vi "Servo Motor Emulator.vi"(10 "Servo Motor Emulator Queue in":refnum<queue>, 11 "Device Manager Queue in":refnum<queue>) -> (0 "error out":errorcluster)   [LabVIEW 2026]
uses:
  support/Message Queue/Message Cluster.ctl
  controls/Servo Controller Private Data.ctl
  support/Message Queue/Enqueue Message (Single).vi
  <vilib>/Utility/error.llb/Error Cluster From Error Code.vi
  <vilib>/ErrorRing/Error Ring.xnode
  support/Message Queue/Message Queue.lvlib
  support/User Event - Stop/User Event - Stop.lvlib
panel:
  in  "RH":dbl
  in  "Temperature":dbl
  out "Position":dbl(knob) scale=0.0..180.0
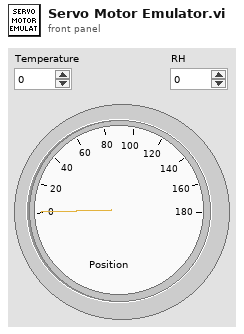
[diagram p1: front panel]
types:
  T1 = typedef "Servo Controller Private Data.ctl" = cluster{"Placeholder":bool}
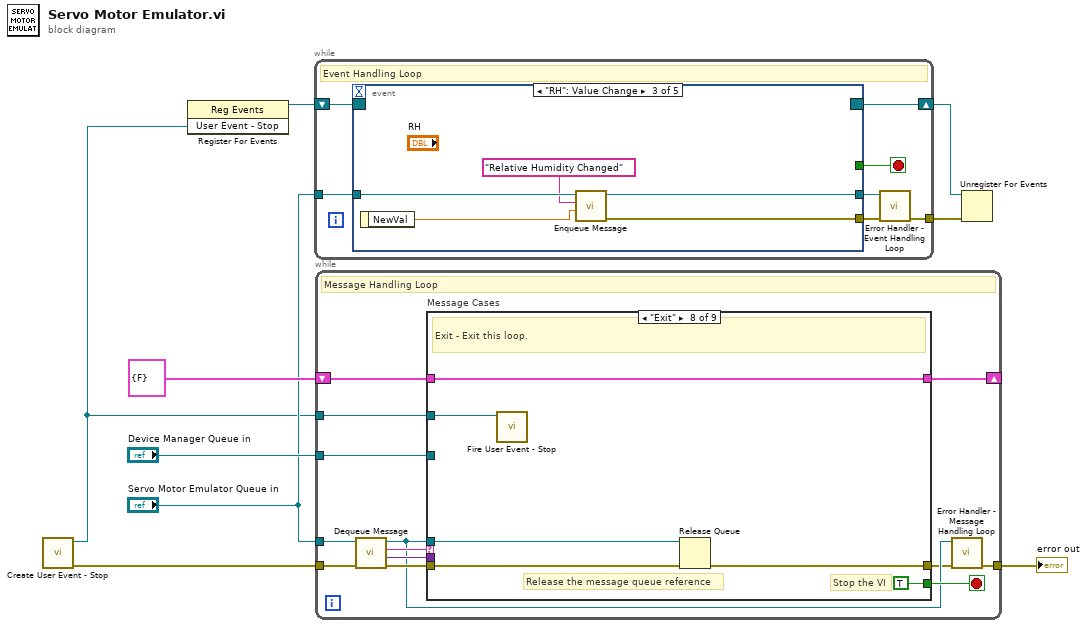
[diagram p0: block diagram]
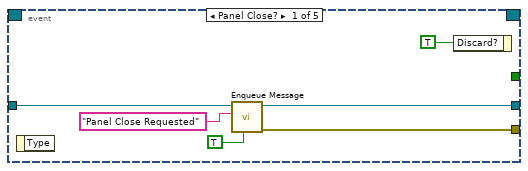
[diagram p2: hidden frame]
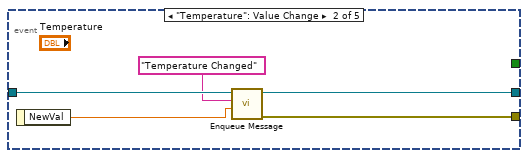
[diagram p3: hidden frame]
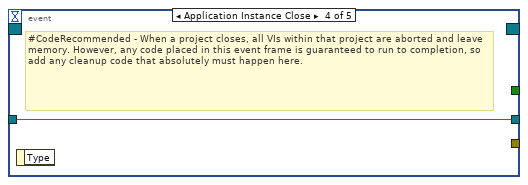
[diagram p4: hidden frame]
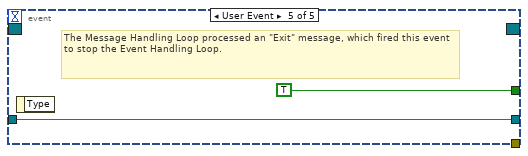
[diagram p5: hidden frame]
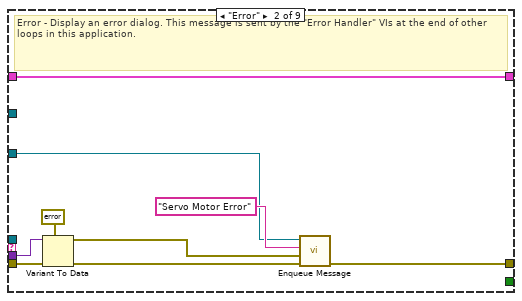
[diagram p7: hidden frame]
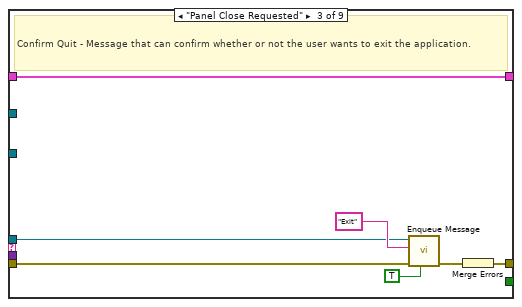
[diagram p8: hidden frame]
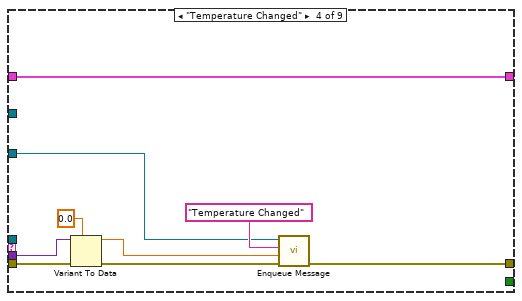
[diagram p9: hidden frame]
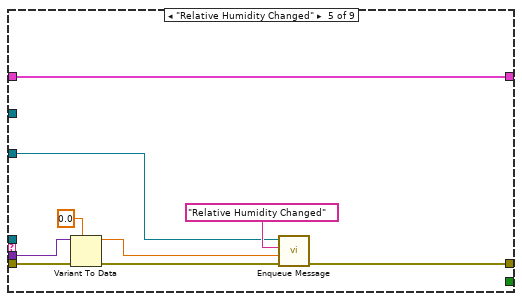
[diagram p10: hidden frame]
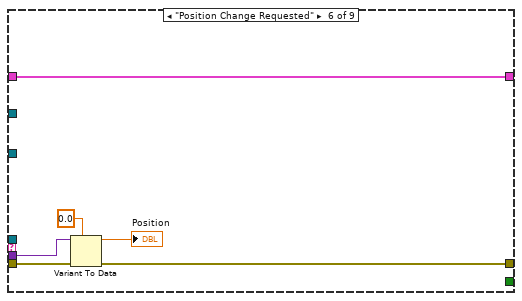
[diagram p11: hidden frame]
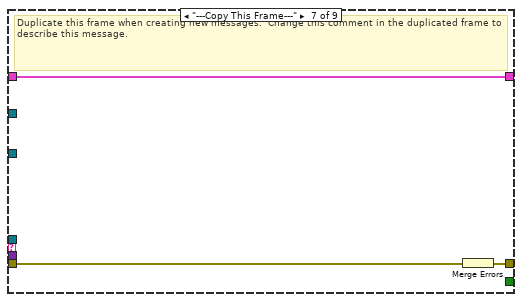
[diagram p12: hidden frame]
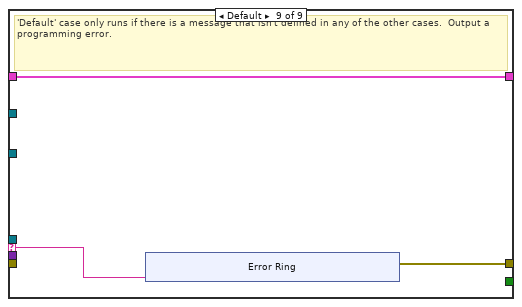
[diagram p13: hidden frame]
diagram:
  n1 = call "Create User Event - Stop.vi"() -> ("error out"=w3:errorcluster, "User Event - Stop"=w1:refnum<user-event>)  [unwired: 10 in]
  n2 = register-events(w1) -> (reference out=w4:refnum<event-registration>)  [unwired: 2 in, 1 out]
  n3 = while {
    tunnel: "Servo Motor Emulator Queue in" -> [w16]
    shift-right: [w14] -> w6
    shift-left: w4 -> [w15]
    tunnel: [w10] -> w5
    stop <- w12 stop-if-true
    # "Event Handling Loop"
    n4 = event shown="[2] \"RH\": Value Change" {
      selector: w15 -> [_ _ _ _ _]
      dyn-events: [_ _ _ _ _] -> w14
      timeout: _ -> [_ _ _ _ _]
      tunnel: [_ _ _ _ TRUE ("Discard?")] -> w12
      tunnel: w16 -> [w21 w27 w32 w33 w35]
      tunnel: [w20 w26 w31 _ _] -> w13
      tunnel: [w19 w25 w30 w33 w35] -> w11
      event Panel Close? {
        n5 = event-data() -> ()  [unwired: 1 in, 1 out]
        n6 = call-poly "Enqueue Message.vi"("Priority Message? (F)"=TRUE, "Message"="Panel Close Requested", "Message Queue"=w21) -> ("error out"=w20:errorcluster, "dup Message Queue"=w19:refnum<queue>)  [unwired: 7 in]
        n7 = event-data("Discard?"=TRUE) -> ()  [unwired: 1 in, 1 out]
      }
      event "Temperature": Value Change {
        n8 = event-data() -> ("NewVal"=w23:dbl)  [unwired: 1 in]
        n9 = call-poly "Enqueue Message.vi"("Message Data"=w23, "Message"="Temperature Changed", "Message Queue"=w27) -> ("error out"=w26:errorcluster, "dup Message Queue"=w25:refnum<queue>)  [unwired: 7 in]
      }
      event "RH": Value Change {
        n10 = event-data() -> ("NewVal"=w28:dbl)  [unwired: 1 in]
        n11 = call-poly "Enqueue Message.vi"("Message Data"=w28, "Message"="Relative Humidity Changed", "Message Queue"=w32) -> ("error out"=w31:errorcluster, "dup Message Queue"=w30:refnum<queue>)  [unwired: 7 in]
      }
      event Application Instance Close {
        # "#CodeRecommended - When a project closes, all VIs within that project are aborted and leave memory. However, any code placed in this event frame is guaranteed to run to completion, so add any cleanup code that absolutely must happen here."
        n12 = event-data() -> ()  [unwired: 1 in, 1 out]
      }
      event User Event {
        # "The Message Handling Loop processed an \"Exit\" message, which fired this event to stop the Event Handling Loop."
        n13 = event-data() -> ()  [unwired: 1 in, 1 out]
      }
    }
    n14 = call "Error Handler - Event Handling Loop.vi"("error in (no error)"=w13, "Message Queue"=w11) -> ("dup error in"=w10:errorcluster)  [unwired: 8 in, 1 out]
  }
  n15 = while {
    tunnel: "Servo Motor Emulator Queue in" -> [w41]
    shift-right: [w47] -> _
    shift-left: T1 {"Placeholder"=FALSE} ("Servo Motor Private Data") -> [w48]
    tunnel: w3 -> [w45]
    tunnel: [w39] -> w9
    tunnel: "Device Manager Queue in" -> [w37]
    tunnel: w1 -> [w36]
    stop <- w46 stop-if-true
    # "Message Handling Loop"
    n16 = call "Dequeue Message.vi"("error in (no error)"=w45, "Message Queue"=w41) -> ("error out"=w44:errorcluster, "Message Data"=w42:variant, "Message"=w43:string, "dup Message Queue"=w40:refnum<queue>)  [unwired: 6 in]
    n17 = case "Message Cases" shown="\"Exit\"" w43 {
      selector: w43 -> [_ _ _ _ _ _ _ _ w100]
      tunnel: w40 -> [_ _ w60 _ _ _ _ w99 _]
      tunnel: w44 -> [w49 w59 w66 w72 w81 w87 w93 w95 _]
      tunnel: [w49 w53 w64 w68 w77 w86 w91 w96 w101] -> w38
      tunnel: w48 -> [w50 w58 w65 w75 w84 w90 w92 w98 w102]
      tunnel: [w50 w58 w65 w75 w84 w90 w92 w98 w102] -> w47
      tunnel: [_ _ _ _ _ _ _ TRUE _] -> w46
      tunnel: w42 -> [_ w57 _ w74 w83 w89 _ _ _]
      tunnel: w37 -> [_ w54 _ w69 w78 _ _ _ _]
      tunnel: w36 -> [_ _ _ _ _ _ _ w94 _]
      frame "Initialize" {
        # "Initialize - All initialization work should take place in this message, since other loops can potentially enqueue messages that execute immediately after this one."
      }
      frame "Error" {
        # "Error - Display an error dialog. This message is sent by the \"Error Handler\" VIs at the end of other loops in this application."
        n18 = Variant To Data(error in=w59, type=errorcluster {"status"=FALSE, "code"=0, "source"=""} ("error constant"), Variant=w57) -> (data=w51:errorcluster, error out=w52:errorcluster)
        n19 = call-poly "Enqueue Message.vi"("error in (no error)"=w52, "Message Data"=w51, "Message"="Servo Motor Error", "Message Queue"=w54) -> ("error out"=w53:errorcluster)  [unwired: 6 in, 1 out]
      }
      frame "Panel Close Requested" {
        # "Confirm Quit - Message that can confirm whether or not the user wants to exit the application."
        n20 = call-poly "Enqueue Message.vi"("Priority Message? (F)"=TRUE, "error in (no error)"=w66, "Message"="Exit", "Message Queue"=w60) -> ("error out"=w63:errorcluster)  [unwired: 6 in, 1 out]
        n21 = Merge Errors(w63) -> (w64:errorcluster)
      }
      frame "Temperature Changed" {
        n22 = Variant To Data(error in=w72, type=0.0 ("Temperature"), Variant=w74) -> (data=w67:dbl, error out=w70:errorcluster)
        n23 = call-poly "Enqueue Message.vi"("error in (no error)"=w70, "Message Data"=w67, "Message"="Temperature Changed", "Message Queue"=w69) -> ("error out"=w68:errorcluster)  [unwired: 6 in, 1 out]
      }
      frame "Relative Humidity Changed" {
        n24 = Variant To Data(error in=w81, type=0.0 ("Temperature"), Variant=w83) -> (data=w76:dbl, error out=w79:errorcluster)
        n25 = call-poly "Enqueue Message.vi"("error in (no error)"=w79, "Message Data"=w76, "Message"="Relative Humidity Changed", "Message Queue"=w78) -> ("error out"=w77:errorcluster)  [unwired: 6 in, 1 out]
      }
      frame "Position Change Requested" {
        n26 = Variant To Data(error in=w87, type=0.0 ("Temperature"), Variant=w89) -> (data=→"Position":dbl, error out=w86:errorcluster)
      }
      frame "---Copy This Frame---" {
        # "Duplicate this frame when creating new messages.  Change this comment in the duplicated frame to describe this message."
        n27 = Merge Errors(w93) -> (w91:errorcluster)
      }
      frame "Exit" {
        # "Stop the VI"
        # "Release the message queue reference"
        # "Exit - Exit this loop."
        n28 = call "Fire User Event - Stop.vi"("User Event - Stop"=w94) -> ()  [unwired: 10 in, 1 out]
        n29 = Release Queue(queue=w99, error in (no error)=w95) -> (error out=w96:errorcluster)  [unwired: 1 in, 2 out]
      }
      frame Default {
        # "'Default' case only runs if there is a message that isn't defined in any of the other cases.  Output a programming error."
        n30 = xnode "Error Ring"("parameter 0"=w100) -> ("error out"=w101:errorcluster)
      }
    }
    n31 = call "Error Handler - Message Handling Loop.vi"("error in (no error)"=w38, "Message Queue"=w40) -> ("dup error in"=w39:errorcluster)  [unwired: 8 in, 1 out]
  }
  "error out" <- w9
  n32 = Unregister For Events(event registration refnum=w6, error in=w5) -> ()  [unwired: 1 out]
